vi "update_attrs.vi"(8 "error in (no error)":errorcluster, 10 "Nested Enqueuers Map":T1(c390), 11 "DAQVoltage in":refnum<class "DAQVoltage.lvclass">) -> (0 "error out":errorcluster, 3 "DAQVoltage out":refnum<class "DAQVoltage.lvclass">)   [LabVIEW 2025, in "DAQVoltage.lvlib" / "DAQVoltage.lvclass"]
uses:
  DAQVoltage.lvclass
  <vilib>/ActorFramework/Message Enqueuer/Message Enqueuer.lvclass
  DAQVoltage.lvclass/DAQVoltage.ctl
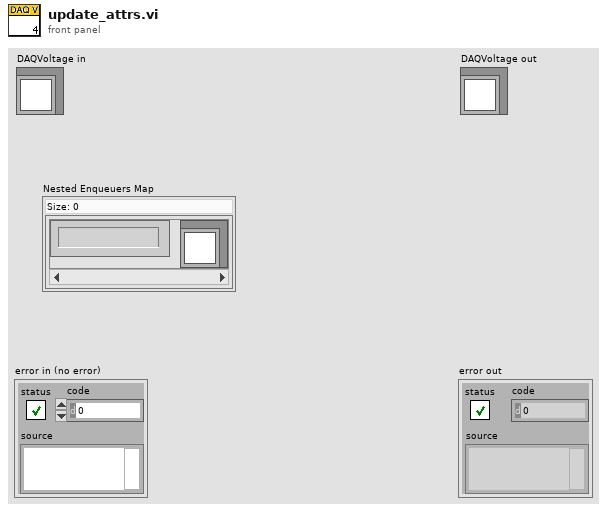
[diagram p1: front panel]
types:
  T1 = map{string, refnum<class "Message Enqueuer.lvclass">}
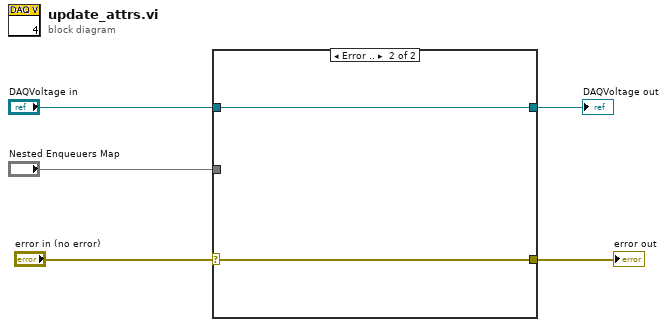
[diagram p0: block diagram]
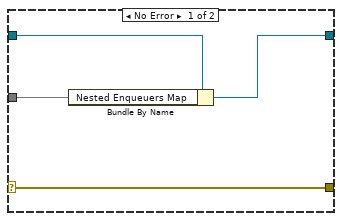
[diagram p2: hidden frame]
diagram:
  n1 = case shown="Error .." "error in (no error)" {
    selector: "error in (no error)" -> [w6 w10]
    tunnel: "DAQVoltage in" -> [w9 w11]
    tunnel: "Nested Enqueuers Map" -> [w8 _]
    tunnel: [w7 w11] -> w3
    tunnel: [w6 w10] -> w1
    frame No Error {
      n2 = Bundle By Name(cluster=w9, "Nested Enqueuers Map"=w8) -> (w7:refnum<class "DAQVoltage.lvclass">)
    }
    frame Error {
    }
  }
  "error out" <- w1
  "DAQVoltage out" <- w3
